vi "PhotonCamera_SetFPSLimit.vi"(9 "FPS":i32, 10 "BaseNTName":string="/photonvision", 11 "CameraName":string) -> (0 "error out":errorcluster)   [LabVIEW 2019, in "PhotonVisionLib.lvlib"]
doc: "Sets the FPS (Frame per second) limit on the camera.\n\nInputs:\n - cameraName -- The nickname of the camera (found in the PhotonVision UI).\n - BaseNTName - string - Base Nework Table name. (Optional. Default: /photonvision )\n - fps -- integer -- The FPS limit to set. Set to -1 for unlimited FPS\n\nOutputs:\n - Error Out -- Contains error information if a Network table ot other error occured."
uses:
  PhotonVisionLib.lvlib
  <vilib>/Rock Robotics/WPI/ThirdParty/JAS_Junk/TrajLib/VI/Util_GetTime_U32.vi
  <vilib>/Rock Robotics/WPI/ThirdParty/JAS_Junk/TrajLib/VI/Util_GetTime_U64.vi
  <vilib>/Rock Robotics/Network Tables/NT Read Integer.vi
  <vilib>/Rock Robotics/Network Tables/NT Write Integer.vi
  <vilib>/Rock Robotics/WPI/ThirdParty/JAS_Junk/TrajLib/Trajectory_Library.lvlib
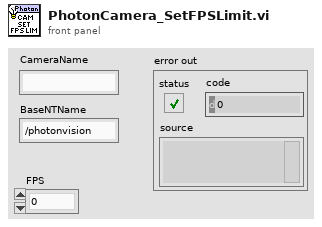
[diagram p1: front panel]
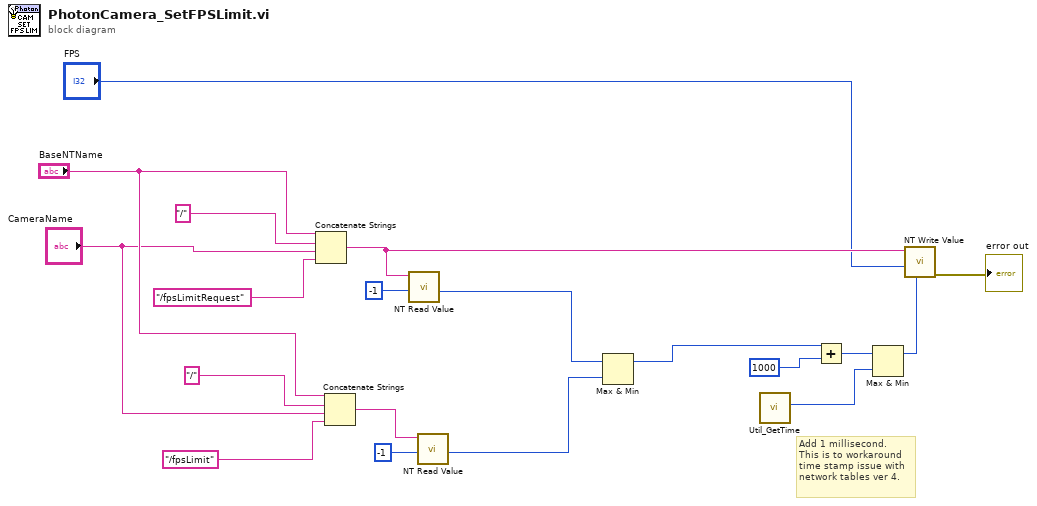
[diagram p0: block diagram]
diagram:
  # "Add 1 millisecond.\nThis is to workaround\ntime stamp issue with\nnetwork tables ver 4."
  n1 = Concatenate Strings("BaseNTName", "/", "CameraName", "/fpsLimitRequest") -> (w12:string)
  n2 = Concatenate Strings("BaseNTName", "/", "CameraName", "/fpsLimit") -> (w6:string)
  n3 = call-poly <vilib>:"NT Read Value.vi"("default value"=i64 -1 ("Default Value"), "name"=w12) -> ("timestamp"=w3:u64)  [unwired: 7 in, 2 out]
  n4 = call-poly <vilib>:"NT Read Value.vi"("default value"=i64 -1 ("Default Value"), "name"=w6) -> ("timestamp"=w2:u64)  [unwired: 7 in, 2 out]
  n5 = Max & Min(x=w3, y=w2) -> (max(x,y)=w1:u64)  [unwired: 1 out]
  n6 = call <vilib>:"Util_GetTime.vi"() -> ("FPGA_Time_MicroSeconds"=w15:u64)  [unwired: 9 in, 2 out]
  n7 = Add(x=w1, y=u64 1000) -> (x+y=w16:u64)
  n8 = Max & Min(x=w16, y=w15) -> (max(x,y)=w13:u64)  [unwired: 1 out]
  n9 = call-poly <vilib>:"NT Write Value.vi"("timestamp"=w13, "value"="FPS", "name"=w12) -> ("error out"=→"error out":errorcluster)  [unwired: 8 in]
